vi "store Listener Command.vi"(0 "Listener Handle in":T1, 5 "Command Handle in":T1, 11 "error in (no error)":errorcluster) -> (4 "Listener Handle out":T1, 15 "error out":errorcluster)   [LabVIEW 2012, in "REx.lvlib" / "Local Listener Session.lvclass"]
uses:
  Local Listener Session.lvclass
  Typedefs/Session Handle.ctl
  Local Listener Session.lvclass/Local Listener Session.ctl
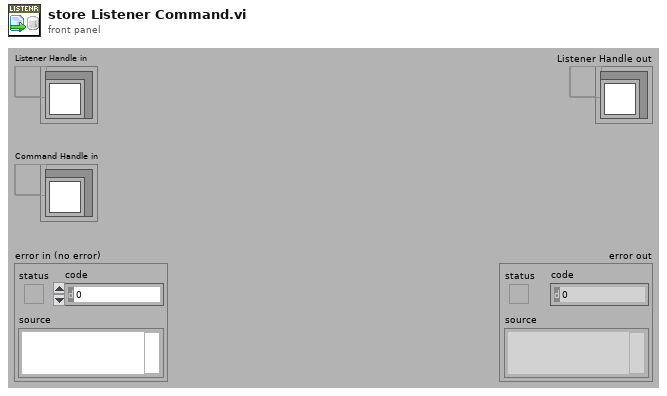
[diagram p1: front panel]
types:
  T1 = typedef "REx.lvlib/Local Listener Session.lvclass/Session Handle.ctl" = refnum<data-value>
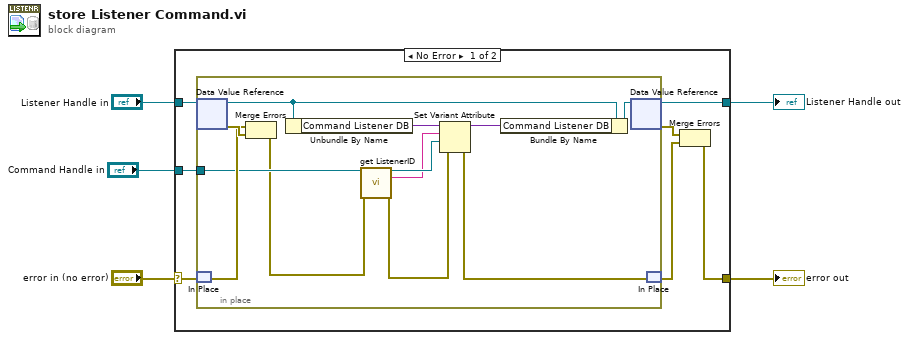
[diagram p0: block diagram]
diagram:
  n1 = case shown="No Error" "error in (no error)" {
    selector: "error in (no error)" -> [w7 w25]
    tunnel: "Listener Handle in" -> [w12 w26]
    tunnel: [w11 w26] -> w4
    tunnel: [w8 w25] -> w3
    tunnel: "Command Handle in" -> [w6 _]
    frame No Error {
      n2 = in-place {
        in-place-border: w6 -> [w17]
        n3 = in-place-dvr #1(w12) -> (w21:refnum<class "Local Listener Session.lvclass">, w24:errorcluster)
        n4 = in-place-match #2(w7) -> (w23:errorcluster)
        n5 = Merge Errors(w23, w24) -> (w15:errorcluster)
        n6 = Unbundle By Name(w21) -> ("Command Listener DB"=w22:variant)
        n7 = call "get ListenerID.vi"("Session Handle in"=w17, "error in (no error)"=w15) -> ("Session Handle out"=w16:T1, "Session Name"=w13:string, "error out"=w14:errorcluster)  [unwired: 11 in]
        n8 = Set Variant Attribute(Variant=w22, name=w13, value=w16, error in=w14) -> (Variant out=w18:variant, error out=w19:errorcluster)  [unwired: 1 out]
        n9 = Bundle By Name(cluster=w21, "Command Listener DB"=w18) -> (w20:refnum<class "Local Listener Session.lvclass">)
        n10 = in-place-dvr #1(w20) -> (w11:T1, w9:errorcluster)
        n11 = in-place-match #2(w19) -> (w10:errorcluster)
      }
      n12 = Merge Errors(w9, w10) -> (w8:errorcluster)
    }
    frame Error {
    }
  }
  "Listener Handle out" <- w4
  "error out" <- w3
